vi "4.7.2.vi"() -> ()   [LabVIEW 2017]
panel:
  out "Случайное целое число":dbl
  in  "OK Button":bool
  in  "stop":bool
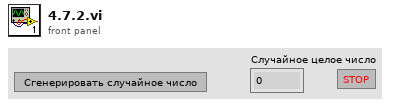
[diagram p1: front panel]
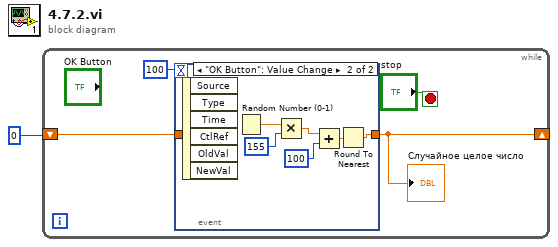
[diagram p0: block diagram]
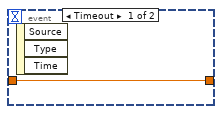
[diagram p2: hidden frame]
diagram:
  n1 = while {
    shift-right: [w2] -> _
    shift-left: 0 -> [w3]
    stop <- "stop" stop-if-true
    n2 = event shown="[1] \"OK Button\": Value Change" {
      selector: _ -> [_ _]
      dyn-events: _ -> [_ _]
      timeout: 100 -> [_ _]
      tunnel: [w6 w8] -> w2
      tunnel: w3 -> [w6 _]
      event Timeout {
        n3 = event-data() -> ()  [unwired: 1 in, 3 out]
      }
      event "OK Button": Value Change {
        n4 = event-data() -> ()  [unwired: 1 in, 6 out]
        n5 = Random Number (0-1)() -> (number: 0 to 1=w11:dbl)
        n6 = Multiply(x=w11, y=155) -> (x*y=w12:dbl)
        n7 = Add(x=w12, y=100) -> (x+y=w7:dbl)
        n8 = Round To Nearest(number=w7) -> (nearest integer value=w8:dbl)
      }
    }
    "Случайное целое число" <- w2
  }
